vi "MQTT Main.vi"() -> ()   [LabVIEW 2017]
uses:
  Q Driver/Controls/IPC-MQTT-Q driver-Q Options.ctl
  Q Driver/Controls/IPC-MQTT-Q driver-En Q Element.ctl
  Controls/MQTT FGV Options.ctl
  Controls/Publish data.ctl
  support/Message Queue/Enqueue Message (Single).vi
  support/Message Queue/Auto Message Queue.lvlib
panel:
  out "Connected":bool
  in  "stop":bool
  out "Message":string[](array[string])
  out "Topic Name":string[](array[string])
  out "error out":errorcluster
  in  "error in (no error)":errorcluster
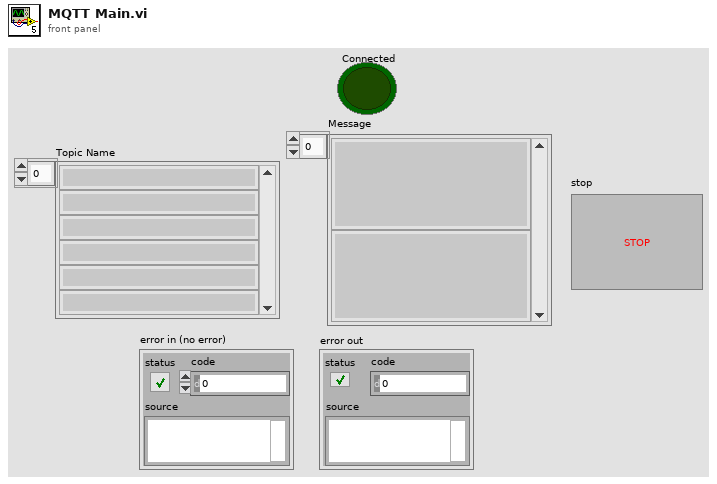
[diagram p1: front panel]
types:
  T1 = cluster{"Topics":string[], "Connected?":bool, "Main VI":refnum<queue>}
  T2 = typedef "IPC-MQTT-Q driver-Q Options.ctl" = enum16{"En Q", "En Q N", "De Q", "Init", "En Q N Stack", "Flush", "Close"}
  T3 = typedef "IPC-MQTT-Q driver-En Q Element.ctl" = cluster{"State":string, "Data":variant}
  T4 = typedef "MQTT FGV Options.ctl" = enum16{"Read", "Subscribe", "Publish", "Get Status", "Connect", "Disconnect"}
  T5 = typedef "Publish data.ctl" = cluster{"Topic":string, "Message":string}
  T6 = typedef "Auto Message Queue.lvlib/All Message Queues.ctl" = cluster{"UI":refnum<queue>}
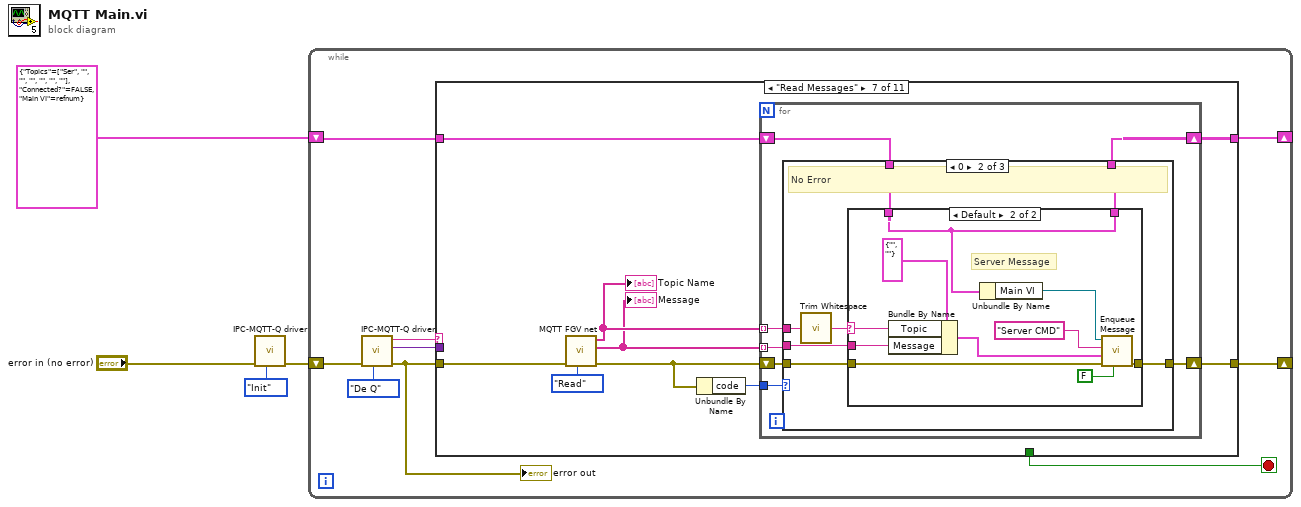
[diagram p0: block diagram]
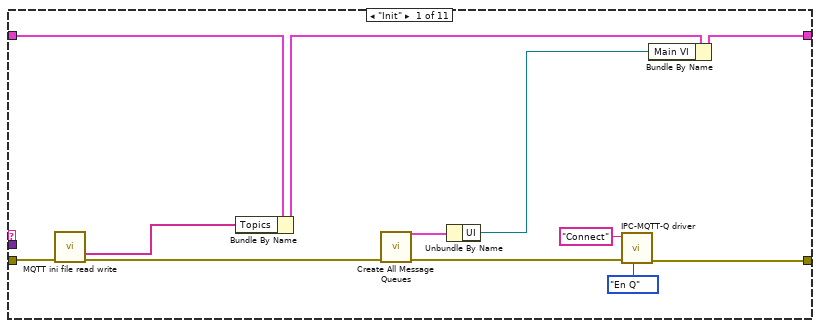
[diagram p2: hidden frame]
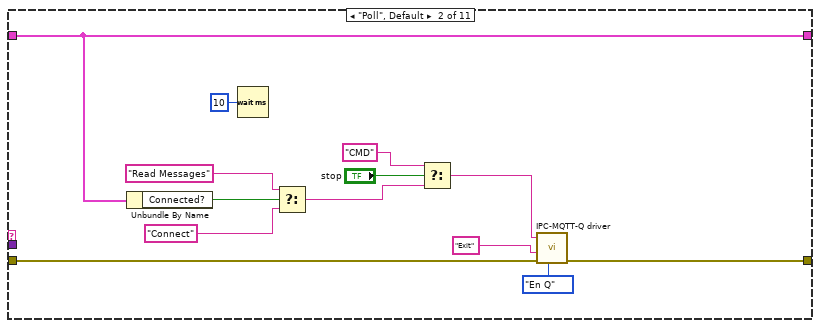
[diagram p3: hidden frame]
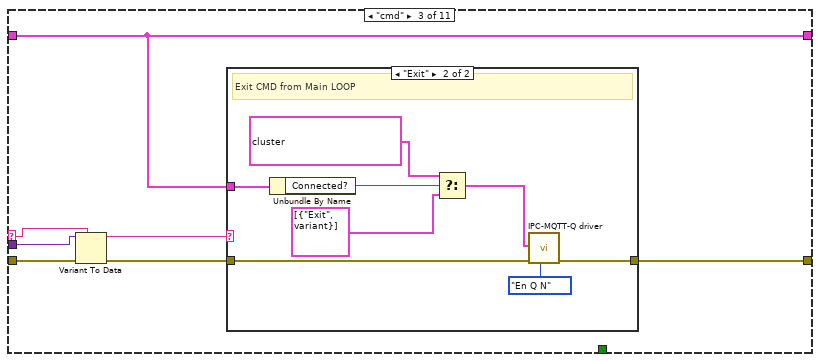
[diagram p4: hidden frame]
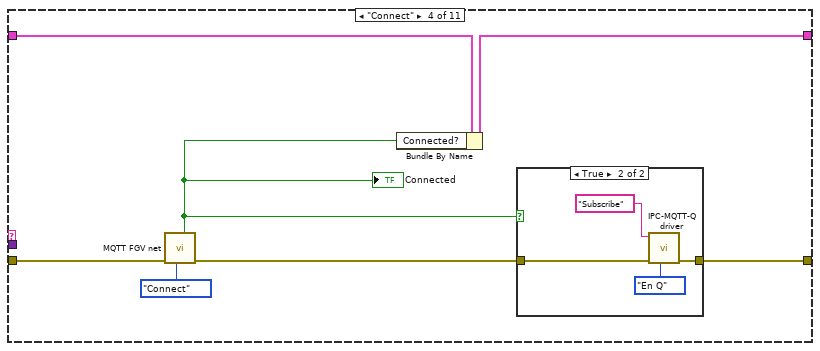
[diagram p6: hidden frame]
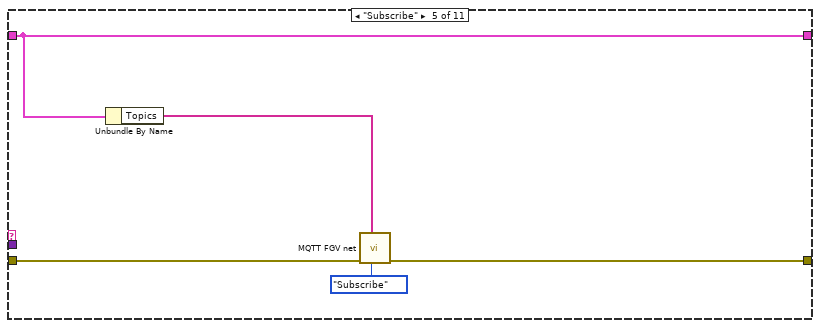
[diagram p8: hidden frame]
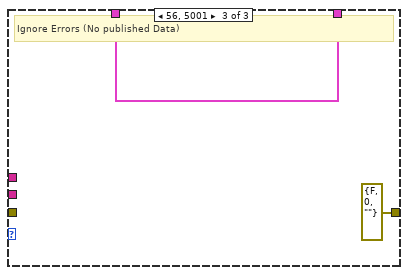
[diagram p12: hidden frame]
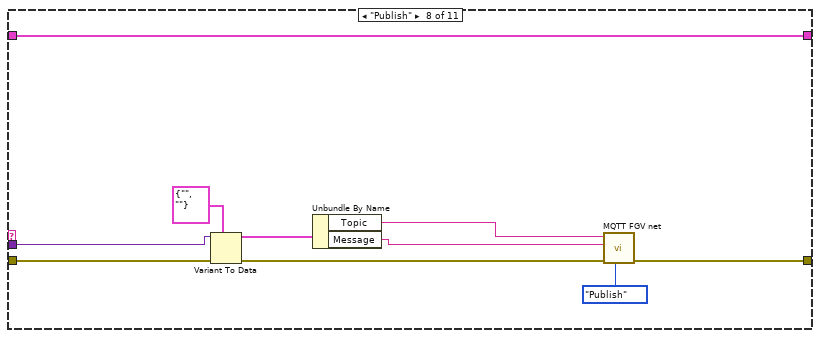
[diagram p13: hidden frame]
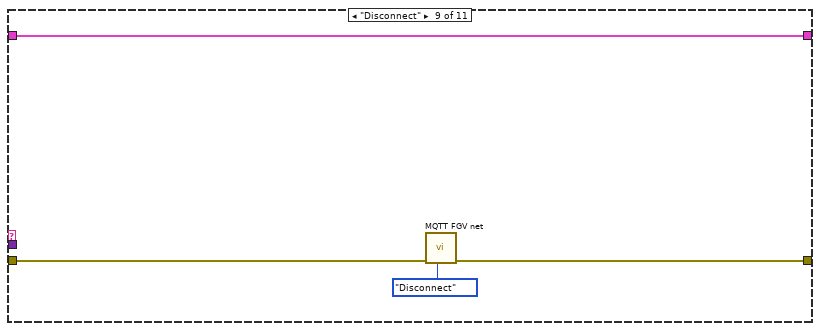
[diagram p14: hidden frame]
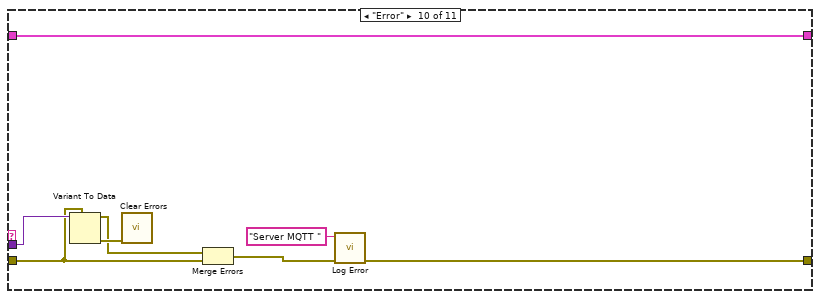
[diagram p15: hidden frame]
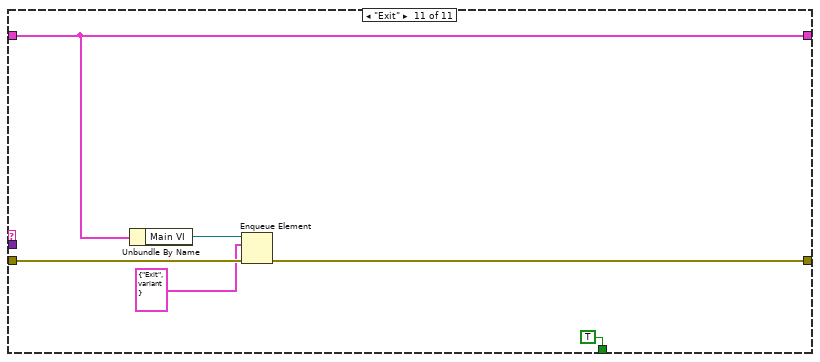
[diagram p16: hidden frame]
diagram:
  n1 = call "IPC-MQTT-Q driver.vi"("Q Options"=IPC-MQTT-Q_driver-Q_Options."Init", "error in (no error)"="error in (no error)") -> ("error out"=w3:errorcluster)  [unwired: 7 in, 2 out]
  n2 = while {
    shift-right: [w11] -> _
    shift-left: w3 -> [w13]
    shift-right: [w6] -> _
    shift-left: T1 {"Topics"=["Ser", "", "", "", "", "", ""], "Connected?"=FALSE, "Main VI"=refnum} -> [w5]
    stop <- w7 stop-if-true
    n3 = call "IPC-MQTT-Q driver.vi"("Q Options"=IPC-MQTT-Q_driver-Q_Options."De Q", "error in (no error)"=w13) -> ("error out"=w12:errorcluster, "Data"=w8:variant, "State"=w9:string)  [unwired: 7 in]
    "error out" <- w12
    n4 = case shown="\"Read Messages\"" w9 {
      selector: w9 -> [_ _ w43 _ _ _ _ _ _ _ _]
      tunnel: w12 -> [w21 w37 w45 w56 w71 w73 w78 w121 w126 w130 w139]
      tunnel: [w15 w36 w39 w60 w68 w73 w81 w116 w124 w133 w138] -> w11
      tunnel: w8 -> [_ _ w44 _ _ _ _ w120 _ w131 _]
      tunnel: [_ _ _ _ _ _ _ _ _ _ TRUE] -> w7
      tunnel: [w19 w30 w41 w59 w67 w72 w79 w122 w125 w134 w137] -> w6
      tunnel: w5 -> [w25 w30 w41 w61 w67 w72 w80 w122 w125 w134 w137]
      frame "Init" {
        n5 = call "MQTT ini file read write.vi"("error in (no error)"=w21) -> ("Topics"=w20:string[], "error out"=w14:errorcluster)  [unwired: 13 in]
        n6 = Bundle By Name(cluster=w25, "Topics"=w20) -> (w24:T1)
        n7 = call "Create All Message Queues.vi"("error in (no error)"=w14) -> ("error out"=w18:errorcluster, "Message Queues out"=w17:T6)  [unwired: 9 in]
        n8 = Unbundle By Name(w17) -> ("UI"=w16:refnum<queue>)
        n9 = call "IPC-MQTT-Q driver.vi"("Q Options"=IPC-MQTT-Q_driver-Q_Options."En Q", "error in (no error)"=w18, "Message"="Connect") -> ("error out"=w15:errorcluster)  [unwired: 6 in, 2 out]
        n10 = Bundle By Name(cluster=w24, "Main VI"=w16) -> (w19:T1)
      }
      frame "Poll", Default {
        n11 = Unbundle By Name(w30) -> ("Connected?"=w29:bool)
        n12 = Wait (ms)(milliseconds to wait=u32 10) -> ()  [unwired: 1 out]
        n13 = Select(t="Read Messages" ("Message"), s=w29, f="Connect" ("Message")) -> (s? t:f=w28:string)
        n14 = Select(t="CMD" ("Message"), s="stop", f=w28) -> (s? t:f=w34:string)
        n15 = call "IPC-MQTT-Q driver.vi"("Q Options"=IPC-MQTT-Q_driver-Q_Options."En Q", "error in (no error)"=w37, "Message Data"="Exit" ("Message"), "Message"=w34) -> ("error out"=w36:errorcluster)  [unwired: 5 in, 2 out]
      }
      frame "cmd" {
        n16 = Variant To Data(error in=w45, type=w43, Variant=w44) -> (data=w42:string, error out=w40:errorcluster)
        n17 = case shown="\"Exit\"" w42 {
          tunnel: w41 -> [_ w54]
          tunnel: w40 -> [w46 w49]
          tunnel: [w46 w48] -> w39
          frame Default {
          }
          frame "Exit" {
            # "Exit CMD from Main LOOP"
            n18 = Unbundle By Name(w54) -> ("Connected?"=w53:bool)
            n19 = Select(t=T3[] [{"State"="Disconnect", "Data"=variant}, {"State"="Exit", "Data"=variant}] ("En Q"), s=w53, f=T3[] [{"State"="Exit", "Data"=variant}]) -> (s? t:f=w47:T3[])
            n20 = call "IPC-MQTT-Q driver.vi"("Q Options"=IPC-MQTT-Q_driver-Q_Options."En Q N", "error in (no error)"=w49, "En Q"=w47) -> ("error out"=w48:errorcluster)  [unwired: 6 in, 2 out]
          }
        }
      }
      frame "Connect" {
        n21 = call "MQTT FGV net.vi"("Options"=MQTT_FGV_Options."Connect", "error in (no error)"=w56) -> ("error out"=w55:errorcluster, "Connected"=w57:bool)  [unwired: 5 in, 3 out]
        "Connected" <- w57
        n22 = Bundle By Name(cluster=w61, "Connected?"=w57) -> (w59:T1)
        n23 = case shown="True" w57 {
          tunnel: w55 -> [w62 w63]
          tunnel: [w62 w65] -> w60
          frame False {
          }
          frame True {
            n24 = call "IPC-MQTT-Q driver.vi"("Q Options"=IPC-MQTT-Q_driver-Q_Options."En Q", "error in (no error)"=w63, "Message"="Subscribe") -> ("error out"=w65:errorcluster)  [unwired: 6 in, 2 out]
          }
        }
      }
      frame "Subscribe" {
        n25 = Unbundle By Name(w67) -> ("Topics"=w70:string[])
        n26 = call "MQTT FGV net.vi"("Options"=MQTT_FGV_Options."Subscribe", "topics"=w70, "error in (no error)"=w71) -> ("error out"=w68:errorcluster)  [unwired: 4 in, 4 out]
      }
      frame "Unsubcribe" {
      }
      frame "Read Messages" {
        n27 = call "MQTT FGV net.vi"("Options"=MQTT_FGV_Options."Read", "error in (no error)"=w78) -> ("error out"=w77:errorcluster, "messagereceived"=w75:string[], "topicrecieved"=w76:string[])  [unwired: 5 in, 2 out]
        "Topic Name" <- w76
        "Message" <- w75
        n28 = Unbundle By Name(w77) -> ("code"=w82:i32)
        n29 = for {
          tunnel: w82 -> [w89]
          tunnel: w76 -> [w84] mode=indexing
          tunnel: w75 -> [w83] mode=indexing
          shift-right: [w86] -> w79
          shift-left: w80 -> [w87]
          shift-right: [w88] -> w81
          shift-left: w77 -> [w85]
          n30 = case shown="0" w89 {
            tunnel: w85 -> [w91 w97 _]
            tunnel: [w91 w96 errorcluster {"status"=FALSE, "code"=0, "source"=""} ("error out")] -> w88
            tunnel: w84 -> [_ w98 _]
            tunnel: w83 -> [_ w95 _]
            tunnel: w87 -> [w90 w93 w111]
            tunnel: [w90 w92 w111] -> w86
            frame Default {
              # "Error While reading Published Message"
            }
            frame 0 {
              # "No Error"
              n31 = call <vilib>:"Trim Whitespace.vi"("string"=w98) -> ("trimmed string"=w94:string)  [unwired: 1 in]
              n32 = case shown="Default" w94 {
                selector: w94 -> [_ w109]
                tunnel: w97 -> [w100 w107]
                tunnel: [w100 w106] -> w96
                tunnel: w95 -> [_ w108]
                tunnel: w93 -> [w99 w103]
                tunnel: [w99 w103] -> w92
                frame "", "Topic" {
                  # "No Published Receieved"
                }
                frame Default {
                  # "Server Message"
                  n33 = Bundle By Name(cluster=T5 {"Topic"="", "Message"=""} ("Cluster"), "Topic"=w109, "Message"=w108) -> (w105:T5)
                  n34 = Unbundle By Name(w103) -> ("Main VI"=w102:refnum<queue>)
                  n35 = call-poly "Enqueue Message.vi"("Priority Message? (F)"=FALSE, "error in (no error)"=w107, "Message Data"=w105, "Message"="Server CMD", "Message Queue"=w102) -> ("error out"=w106:errorcluster)  [unwired: 5 in, 1 out]
                }
              }
            }
            frame 56, 5001 {
              # "Ignore Errors (No published Data)"
            }
          }
        }
      }
      frame "Publish" {
        n36 = Variant To Data(error in=w121, type=T5 {"Topic"="", "Message"=""} ("Cluster"), Variant=w120) -> (data=w118:T5, error out=w117:errorcluster)
        n37 = Unbundle By Name(w118) -> ("Topic"=w114:string, "Message"=w113:string)
        n38 = call "MQTT FGV net.vi"("Options"=MQTT_FGV_Options."Publish", "error in (no error)"=w117, "Message"=w113, "Topic"=w114) -> ("error out"=w116:errorcluster)  [unwired: 3 in, 4 out]
      }
      frame "Disconnect" {
        n39 = call "MQTT FGV net.vi"("Options"=MQTT_FGV_Options."Disconnect", "error in (no error)"=w126) -> ("error out"=w124:errorcluster)  [unwired: 5 in, 4 out]
      }
      frame "Error" {
        n40 = Variant To Data(type=w130, Variant=w131) -> (data=w127:errorcluster, error out=w129:errorcluster)  [unwired: 1 in]
        n41 = call <vilib>:"Clear Errors.vi"("error in (no error)"=w129) -> ()  [unwired: 5 in, 2 out]
        n42 = Merge Errors(w127, w130) -> (w128:errorcluster)
        n43 = call "Log Error.vi"("error in (no error)"=w128, "VI Name"="Server MQTT ") -> ("error out"=w133:errorcluster)  [unwired: 9 in]
      }
      frame "Exit" {
        n44 = Unbundle By Name(w137) -> ("Main VI"=w136:refnum<queue>)
        n45 = Enqueue Element(queue=w136, element=T3 {"State"="Exit", "Data"=variant}, error in (no error)=w139) -> (error out=w138:errorcluster)  [unwired: 1 in, 2 out]
      }
    }
  }
